vi "CTRE_SensoredMecanum_Servo_Turn_Imu.vi"(5 "Angle Tolerance":dbl format="%#_13g", 6 "Servo Params":T1, 7 "PigeonIMU":T8={"DeviceStatus"={"status"=FALSE, "code"=0, "source"=""}, "Device Number"=0, "Type"=352321536, "Device ID"=0, "Handle"=0, "UsageFrame"=0, "Library Path"=path ""} {"Type" items=["CAN"=352321536, "TalonSRX"=33554432]}, 9 "Set Angle":dbl format="%#_13g", 10 "Talon SRX Control Mode":T10, 11 "Sensored Mecanum":T2={"Sensored Gearbox Front Left"={"Smart Motor Controller"={"DeviceStatus"={"status"=FALSE, "code"=0, "source"=""}, "Type"=enum."PWM", "PWM"={"PWM Channel"=enum."PWM 1", "DeadBand"={"Name"="", "maxPositivePwm"=0, "minPositivePwm"=0, "centerPwm"=0, "maxNegativePwm"=0, "minNegativePwm"=0, "angularRange"=0}}, "CAN"={"Device Number"=0, "SetOutput VI Ref"=variant(enum8{"Percent VBus", "Current", "Speed", "Position", "Voltage"} enum."Percent VBus"), "GetOutput VI Ref"=variant(refnum<k1> refnum), "Enable VI Ref"=variant(dbl 12.0), "Disable VI Ref"=variant(enum8{"Percent VBus", "Speed", "Position", "Slave", "Unchanged / Invalid", "Voltage Compensation", "Current", "Motion Profile"} enum."Percent VBus"), "Data"=variant}, "Invert"=FALSE}, "Invert"=FALSE, "Gear Ratio"=0.0}, "Sensored Gearbox Front Right "={"Smart Motor Controller"={"DeviceStatus"={"status"=FALSE, "code"=0, "source"=""}, "Type"=enum."PWM", "PWM"={"PWM Channel"=enum."PWM 1", "DeadBand"={"Name"="", "maxPositivePwm"=0, "minPositivePwm"=0, "centerPwm"=0, "maxNegativePwm"=0, "minNegativePwm"=0, "angularRange"=0}}, "CAN"={"Device Number"=0, "SetOutput VI Ref"=variant(enum8{"Percent VBus", "Current", "Speed", "Position", "Voltage"} enum."Percent VBus"), "GetOutput VI Ref"=variant(refnum<k1> refnum), "Enable VI Ref"=variant(dbl 12.0), "Disable VI Ref"=variant(enum8{"Percent VBus", "Speed", "Position", "Slave", "Unchanged / Invalid", "Voltage Compensation", "Current", "Motion Profile"} enum."Percent VBus"), "Data"=variant}, "Invert"=FALSE}, "Invert"=FALSE, "Gear Ratio"=0.0}, "Sensored Gearbox Back Left "={"Smart Motor Controller"={"DeviceStatus"={"status"=FALSE, "code"=0, "source"=""}, "Type"=enum."PWM", "PWM"={"PWM Channel"=enum."PWM 1", "DeadBand"={"Name"="", "maxPositivePwm"=0, "minPositivePwm"=0, "centerPwm"=0, "maxNegativePwm"=0, "minNegativePwm"=0, "angularRange"=0}}, "CAN"={"Device Number"=0, "SetOutput VI Ref"=variant(enum8{"Percent VBus", "Current", "Speed", "Position", "Voltage"} enum."Percent VBus"), "GetOutput VI Ref"=variant(refnum<k1> refnum), "Enable VI Ref"=variant(dbl 12.0), "Disable VI Ref"=variant(enum8{"Percent VBus", "Speed", "Position", "Slave", "Unchanged / Invalid", "Voltage Compensation", "Current", "Motion Profile"} enum."Percent VBus"), "Data"=variant}, "Invert"=FALSE}, "Invert"=FALSE, "Gear Ratio"=0.0}, "Sensored Gearbox Back Right  "={"Smart Motor Controller"={"DeviceStatus"={"status"=FALSE, "code"=0, "source"=""}, "Type"=enum."PWM", "PWM"={"PWM Channel"=enum."PWM 1", "DeadBand"={"Name"="", "maxPositivePwm"=0, "minPositivePwm"=0, "centerPwm"=0, "maxNegativePwm"=0, "minNegativePwm"=0, "angularRange"=0}}, "CAN"={"Device Number"=0, "SetOutput VI Ref"=variant(enum8{"Percent VBus", "Current", "Speed", "Position", "Voltage"} enum."Percent VBus"), "GetOutput VI Ref"=variant(refnum<k1> refnum), "Enable VI Ref"=variant(dbl 12.0), "Disable VI Ref"=variant(enum8{"Percent VBus", "Speed", "Position", "Slave", "Unchanged / Invalid", "Voltage Compensation", "Current", "Motion Profile"} enum."Percent VBus"), "Data"=variant}, "Invert"=FALSE}, "Invert"=FALSE, "Gear Ratio"=0.0}, "Wheel Radius"=0.0, "Distance Between Wheels"=0.0}) -> (0 "At Target":bool, 2 "Sensored Mecanum Servo Turn IMU":T11 {"PigeonIMU"."Type" items=["CAN"=352321536, "TalonSRX"=33554432]}, 3 "Sensored Mecanum":T2={"Sensored Gearbox Front Left"={"Smart Motor Controller"={"DeviceStatus"={"status"=FALSE, "code"=0, "source"=""}, "Type"=enum."PWM", "PWM"={"PWM Channel"=enum."PWM 1", "DeadBand"={"Name"="", "maxPositivePwm"=0, "minPositivePwm"=0, "centerPwm"=0, "maxNegativePwm"=0, "minNegativePwm"=0, "angularRange"=0}}, "CAN"={"Device Number"=0, "SetOutput VI Ref"=variant(enum8{"Percent VBus", "Current", "Speed", "Position", "Voltage"} enum."Percent VBus"), "GetOutput VI Ref"=variant(refnum<k1> refnum), "Enable VI Ref"=variant(dbl 12.0), "Disable VI Ref"=variant(enum8{"Percent VBus", "Speed", "Position", "Slave", "Unchanged / Invalid", "Voltage Compensation", "Current", "Motion Profile"} enum."Percent VBus"), "Data"=variant}, "Invert"=FALSE}, "Invert"=FALSE, "Gear Ratio"=0.0}, "Sensored Gearbox Front Right "={"Smart Motor Controller"={"DeviceStatus"={"status"=FALSE, "code"=0, "source"=""}, "Type"=enum."PWM", "PWM"={"PWM Channel"=enum."PWM 1", "DeadBand"={"Name"="", "maxPositivePwm"=0, "minPositivePwm"=0, "centerPwm"=0, "maxNegativePwm"=0, "minNegativePwm"=0, "angularRange"=0}}, "CAN"={"Device Number"=0, "SetOutput VI Ref"=variant(enum8{"Percent VBus", "Current", "Speed", "Position", "Voltage"} enum."Percent VBus"), "GetOutput VI Ref"=variant(refnum<k1> refnum), "Enable VI Ref"=variant(dbl 12.0), "Disable VI Ref"=variant(enum8{"Percent VBus", "Speed", "Position", "Slave", "Unchanged / Invalid", "Voltage Compensation", "Current", "Motion Profile"} enum."Percent VBus"), "Data"=variant}, "Invert"=FALSE}, "Invert"=FALSE, "Gear Ratio"=0.0}, "Sensored Gearbox Back Left "={"Smart Motor Controller"={"DeviceStatus"={"status"=FALSE, "code"=0, "source"=""}, "Type"=enum."PWM", "PWM"={"PWM Channel"=enum."PWM 1", "DeadBand"={"Name"="", "maxPositivePwm"=0, "minPositivePwm"=0, "centerPwm"=0, "maxNegativePwm"=0, "minNegativePwm"=0, "angularRange"=0}}, "CAN"={"Device Number"=0, "SetOutput VI Ref"=variant(enum8{"Percent VBus", "Current", "Speed", "Position", "Voltage"} enum."Percent VBus"), "GetOutput VI Ref"=variant(refnum<k1> refnum), "Enable VI Ref"=variant(dbl 12.0), "Disable VI Ref"=variant(enum8{"Percent VBus", "Speed", "Position", "Slave", "Unchanged / Invalid", "Voltage Compensation", "Current", "Motion Profile"} enum."Percent VBus"), "Data"=variant}, "Invert"=FALSE}, "Invert"=FALSE, "Gear Ratio"=0.0}, "Sensored Gearbox Back Right  "={"Smart Motor Controller"={"DeviceStatus"={"status"=FALSE, "code"=0, "source"=""}, "Type"=enum."PWM", "PWM"={"PWM Channel"=enum."PWM 1", "DeadBand"={"Name"="", "maxPositivePwm"=0, "minPositivePwm"=0, "centerPwm"=0, "maxNegativePwm"=0, "minNegativePwm"=0, "angularRange"=0}}, "CAN"={"Device Number"=0, "SetOutput VI Ref"=variant(enum8{"Percent VBus", "Current", "Speed", "Position", "Voltage"} enum."Percent VBus"), "GetOutput VI Ref"=variant(refnum<k1> refnum), "Enable VI Ref"=variant(dbl 12.0), "Disable VI Ref"=variant(enum8{"Percent VBus", "Speed", "Position", "Slave", "Unchanged / Invalid", "Voltage Compensation", "Current", "Motion Profile"} enum."Percent VBus"), "Data"=variant}, "Invert"=FALSE}, "Invert"=FALSE, "Gear Ratio"=0.0}, "Wheel Radius"=0.0, "Distance Between Wheels"=0.0})   [LabVIEW 2016]
uses:
  <vilib>/Rock Robotics/WPI/ThirdParty/CanMotor/CTRLib-LV-TalonSRX/CTRE_CANTalonSRX_ControlMode.ctl
  <vilib>/Rock Robotics/WPI/ThirdParty/Sensors/Pigeon IMU/CTRE_PigeonIMU_DeviceRef.ctl
  <vilib>/Rock Robotics/WPI/ThirdParty/Sensors/Pigeon IMU/CTRE_PigeonIMU_ConnectionType.ctl
  <vilib>/Rock Robotics/WPI/ThirdParty/CanMotor/CTRLib-LV-TalonSRX/Framework/SensoredMecanum.ctl
  <vilib>/Rock Robotics/WPI/ThirdParty/CanMotor/CTRLib-LV-TalonSRX/Framework/SensoredGearbox.ctl
  <vilib>/Rock Robotics/WPI/MotorControl/WPI_MotorControlDeviceRef.ctl
  <vilib>/Rock Robotics/WPI/MotorControl/WPI_MotorControlType.ctl
  <vilib>/Rock Robotics/SystemInterfaces/DIO/FPGA_DIOPWMChannel.ctl
  <vilib>/Rock Robotics/WPI/PWM/WPI_PWMDeadband.ctl
  <vilib>/Rock Robotics/WPI/ThirdParty/CanMotor/CTRLib-LV-TalonSRX/Framework/ServoParams.ctl
  <vilib>/Rock Robotics/WPI/ThirdParty/Sensors/Pigeon IMU/CTRE_PigeonIMU_GetRawGyro.vi
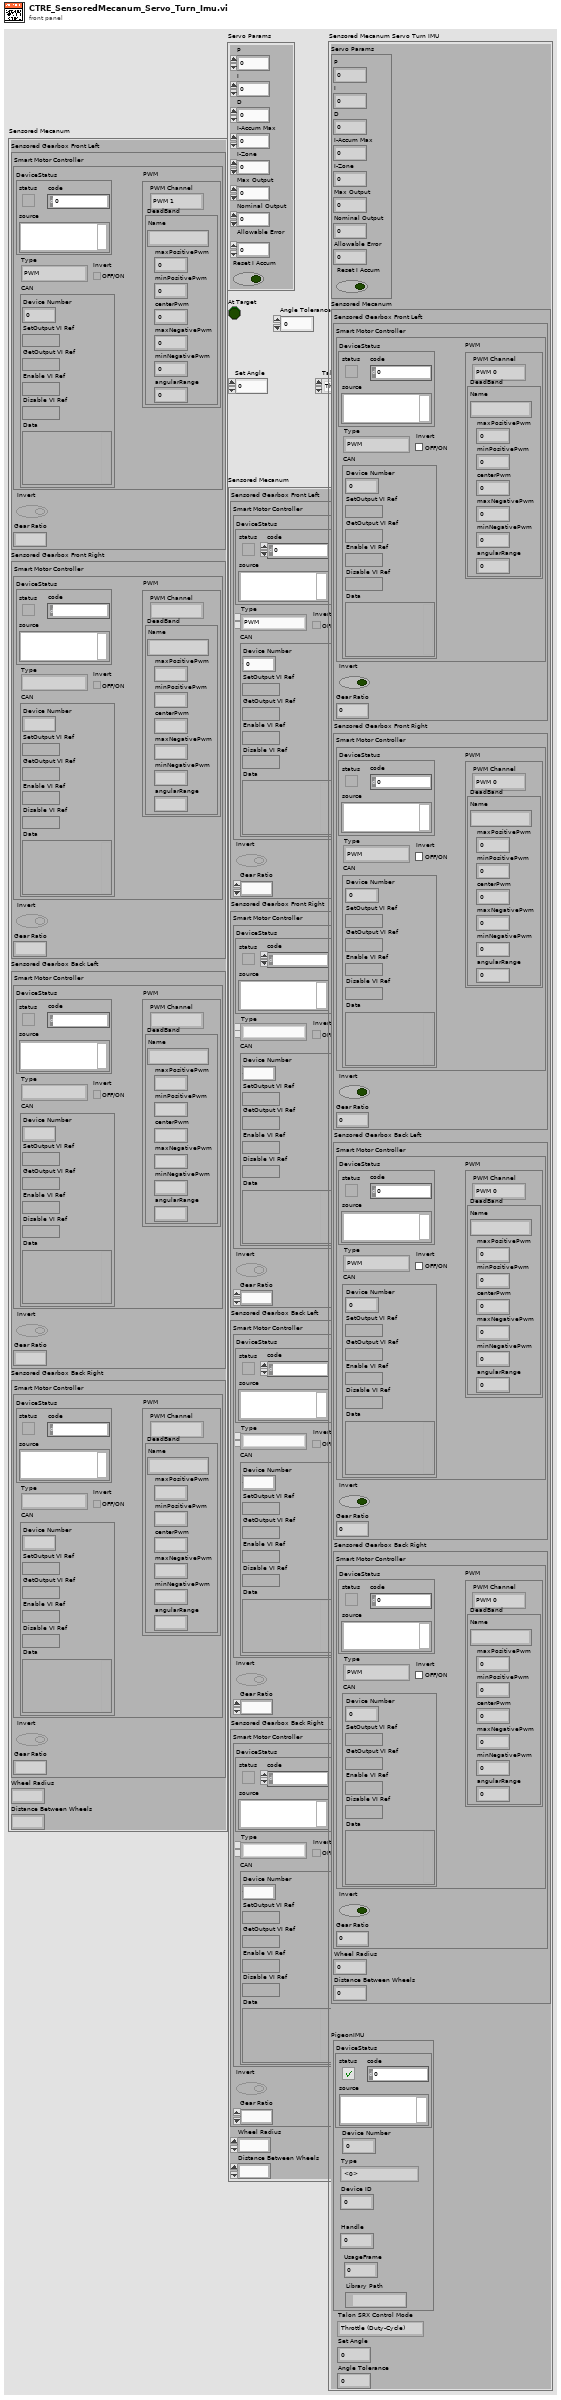
[diagram p1: front panel]
types:
  T1 = typedef "ServoParams.ctl" = cluster{"P":dbl, "I":dbl, "D":dbl, "I-Accum Max":dbl, "I-Zone":dbl, "Max Output":dbl, "Nominal Output":dbl, "Allowable Error":dbl, "Reset I Accum":bool}
  T2 = typedef "SensoredMecanum.ctl" = cluster{"Sensored Gearbox Front Left":T3, "Sensored Gearbox Front Right ":T3, "Sensored Gearbox Back Left ":T3, "Sensored Gearbox Back Right  ":T3, "Wheel Radius":dbl, "Distance Between Wheels":dbl}
  T3 = typedef "SensoredGearbox.ctl" = cluster{"Smart Motor Controller":T4, "Invert":bool, "Gear Ratio":dbl}
  T4 = typedef "WPI_MotorControlDeviceRef.ctl" = cluster{"DeviceStatus":errorcluster, "Type":T5, "PWM":cluster{"PWM Channel":T6, "DeadBand":T7}, "CAN":cluster{"Device Number":u8, "SetOutput VI Ref":variant, "GetOutput VI Ref":variant, "Enable VI Ref":variant, "Disable VI Ref":variant, "Data":variant}, "Invert":bool}
  T5 = typedef "WPI_MotorControlType.ctl" = enum16{"PWM", "CAN"}
  T6 = typedef "FPGA_DIOPWMChannel.ctl" = enum8{"PWM 0", "PWM 1", "PWM 2", "PWM 3", "PWM 4", "PWM 5", "PWM 6", "PWM 7", "PWM 8", "PWM 9", "PWM MXP 0", "PWM MXP 1", "PWM MXP 2", "PWM MXP 3", "PWM MXP 4", "PWM MXP 5", "PWM MXP 6", "PWM MXP 7", "PWM MXP 8", "PWM MXP 9", "Invalid"}
  T7 = typedef "WPI_PWMDeadband.ctl" = cluster{"Name":string, "maxPositivePwm":i32, "minPositivePwm":i32, "centerPwm":i32, "maxNegativePwm":i32, "minNegativePwm":i32, "angularRange":u16}
  T8 = typedef "CTRE_PigeonIMU_DeviceRef.ctl" = cluster{"DeviceStatus":errorcluster, "Device Number":u8, "Type":T9, "Device ID":u32, "Handle":u64, "UsageFrame":u32, "Library Path":path}
  T9 = typedef "CTRE_PigeonIMU_ConnectionType.ctl" = u32
  T10 = typedef "CTRE_CANTalonSRX_ControlMode.ctl" = enum16{"Throttle (Duty-Cycle)", "Position Closed-Loop", "Velocity Closed-Loop", "Current Closed-Loop", "Voltage Compensation", "Slave Follower", "Motion Profile", "Motion Magic"}
  T11 = cluster{"Servo Params":T1, "Sensored Mecanum":T2, "PigeonIMU":T8, "Talon SRX Control Mode":T10, "Set Angle":dbl, "Angle Tolerance":dbl}
  T12 = cluster{"X":dbl, "Y":dbl, "Z":dbl, "Magnitude":dbl}
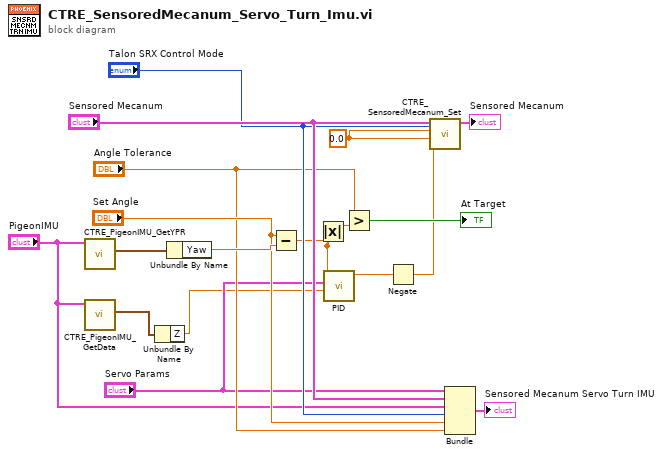
[diagram p0: block diagram]
diagram:
  w15 = 0.0 ("Forward")
  n1 = call <vilib>:"CTRE_PigeonIMU_GetYPR.vi"("PigeonIMUDevRef"="PigeonIMU") -> ("Yaw Pitch Roll"=w18:cluster{"Yaw":dbl, "Pitch":dbl, "Roll":dbl})  [unwired: 8 in, 2 out]
  n2 = call-poly <vilib>:"CTRE_PigeonIMU_GetData.vi"("PigeonIMUDevRef"="PigeonIMU") -> ("Gyro DPS"=w6:T12)  [unwired: 8 in, 2 out]
  n3 = Unbundle By Name(w6) -> ("Z"=w3:dbl)
  n4 = Unbundle By Name(w18) -> ("Yaw"=w17:dbl)
  n5 = Subtract(x="Set Angle", y=w17) -> (x-y=w11:dbl)
  n6 = Absolute Value(x=w11) -> (abs(x)=w10:dbl)
  n7 = call <vilib>:"PID.vi"("Sensor Derivative"=w3, "Servo Params"="Servo Params", "Error"=w11) -> ("Out"=w2:dbl)  [unwired: 8 in]
  n8 = Greater?(x="Angle Tolerance", y=w10) -> (0:→"At Target":bool)
  n9 = Negate(x=w2) -> (-x=w5:dbl)
  n10 = call <vilib>:"CTRE_SensoredMecanum_Set.vi"("Talon SRX Control Mode"="Talon SRX Control Mode", "Turn"=w5, "Strafe"=w15, "Forward"=w15, "Sensored Mecanum"="Sensored Mecanum") -> ("Sensored Mecanum"=→"Sensored Mecanum":T2)  [unwired: 5 in, 1 out]
  n11 = Bundle("Servo Params"="Servo Params", "Sensored Mecanum"="Sensored Mecanum", "PigeonIMU"="PigeonIMU", "Talon SRX Control Mode"="Talon SRX Control Mode", "Set Angle"="Set Angle", "Angle Tolerance"="Angle Tolerance") -> (→"Sensored Mecanum Servo Turn IMU":T11)  [unwired: 1 in]
